vi "DB.indexrange_lua.vi"(5 "LuaVIEW reference":T1) -> (15 "error out":errorcluster)   [LabVIEW 2012]
doc: "Read an index range of values and their corresponding timestamps from a tag's log. Use an index of zero to read from the start of the tag log. By reading a moderate number of values and incrementing the index in a loop, it is possible to efficiently process more values than will fit in memory. To process all values in a log, first use <code>DB.logsize</code> to determine the number of logged values.\n\nBeware that this function may take a while to complete. Because of contention this can happen even when the amount of data being queried is small.\nParameters:\nobj:db, database object.\nstr:tag, name of the tag.\nnum:index, starting index to read from. May not exceed the log size minus the number values being read.\nnum:number, number of values (points or strings) to read as of the specified index.\nResults:\ntab:values, number values, in case of a number tag, or string values, in case of a string tag.\ntab:times, timestamps of the read values.\nErrors:\nTag does not exist.\nDatabases module not initialised.\nCannot read more than \"max points\" values."
uses:
  luaview/typedefs/t_LuaVIEW Reference.ctl
  luaview/subvis/private/LuaVIEW Pull (string).vi
  luaview/subvis/private/LuaVIEW Pull (number).vi
  luaview/subvis/private/LuaVIEW Pull (I32).vi
  luaview/subvis/private/re_LuaVIEW Push (flat data).vi
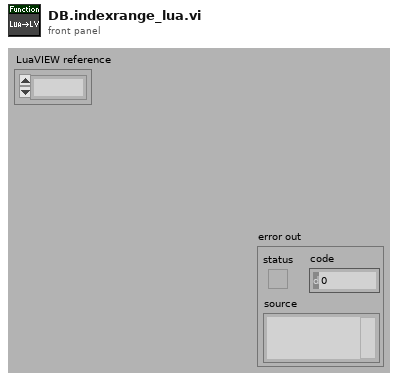
[diagram p1: front panel]
types:
  T1 = typedef "t_LuaVIEW Reference.ctl" = refnum<k1>
  T2 = typedef "t_DataLog Database Info Pane.ctl" = refnum<vi>
  T3 = typedef "t_DataLog Tag Config.ctl" = cluster{"name":string, "unit":string, "temporal":T4, "value":T5, "index":i32, "capacity":i32, "is meta?":bool, "mincapacity":i32, "deadband":dbl, "limit delay":dbl, "format":T6, "precision":u8, "undefine":bool, "update":bool, "update period":u16, "expression":string, "description":string, "logging algorithm":T7, "logging parameters":dbl[]}
  T4 = typedef "t_DataLog Temporal Types.ctl" = enum16{"set&hold", "sample", "event"}
  T5 = typedef "t_DataLog Value Types.ctl" = enum16{"number", "string"}
  T6 = typedef "t_DataLog Numerical Format.ctl" = enum8{"fractional", "exponential", "engineering"}
  T7 = typedef "t_DataLog Logging Algorithms.ctl" = enum16{"nothing", "changes", "everything", "every Nth", "time threshold", "value threshold + prior", "t or v threshold", "t or v threshold + prior"}
  T8 = typedef "t_DataLog Point.ctl" = cluster{"time":dbl, "value":dbl}
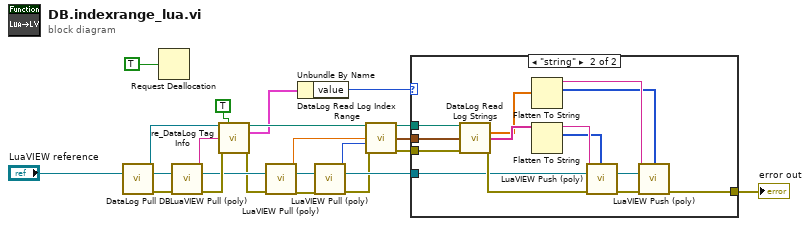
[diagram p0: block diagram]
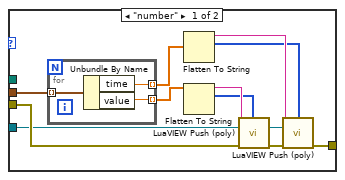
[diagram p2: hidden frame]
diagram:
  n1 = call "DataLog Pull DB.vi"("LuaVIEW reference in"="LuaVIEW reference") -> ("database info"=w1:T2, "LuaVIEW reference out"=w4:T1, "error out"=w2:errorcluster)  [unwired: 12 in]
  n2 = Request Deallocation(TRUE ("flag")) -> ()
  n3 = call-poly "LuaVIEW Pull (poly).vi"("LuaVIEW reference in"=w4, "error in (no error)"=w2) -> ("string"=w5:string, "LuaVIEW reference out"=w9:T1, "error out"=w11:errorcluster)  [unwired: 11 in]
  n4 = call "re_DataLog Tag Info.vi"("database ref (use name)"=w1, "flush? (false)"=TRUE, "tag"=w5, "error in (no error)"=w11) -> ("tag log directory"=w7:path, "tag config"=w6:T3, "error out"=w8:errorcluster)  [unwired: 8 in, 1 out]
  n5 = call-poly "LuaVIEW Pull (poly).vi"("LuaVIEW reference in"=w9, "error in (no error)"=w8) -> ("number"=w14:dbl, "LuaVIEW reference out"=w22:T1, "error out"=w23:errorcluster)  [unwired: 11 in]
  n6 = Unbundle By Name(w6) -> ("value"=w21:T5)
  n7 = call-poly "LuaVIEW Pull (poly).vi"("LuaVIEW reference in"=w22, "error in (no error)"=w23) -> ("I32"=w15:i32, "LuaVIEW reference out"=w20:T1, "error out"=w16:errorcluster)  [unwired: 11 in]
  n8 = call "DataLog Read Log Index Range.vi"("tag log directory"=w7, "log index"=w14, "number of points"=w15, "error in (no error)"=w16) -> ("dup tag log directory"=w19:path, "range of points"=w18:T8[], "error out"=w17:errorcluster)  [unwired: 9 in]
  n9 = case shown="\"string\"" w21 {
    tunnel: w17 -> [w28 w52]
    tunnel: w18 -> [w26 w51]
    tunnel: w19 -> [_ w50]
    tunnel: w20 -> [w27 w48]
    tunnel: [w29 w39] -> w13
    frame "number" {
      n10 = for {
        tunnel: w26 -> [w38] mode=indexing
        tunnel: [w37] -> w25 mode=indexing
        tunnel: [w36] -> w24 mode=indexing
        n11 = Unbundle By Name(w38) -> ("time"=w36:dbl, "value"=w37:dbl)
      }
      n12 = Flatten To String(anything=w24) -> (data string=w31:string, type string=w30:i16[])  [unwired: 3 in, 1 out]
      n13 = Flatten To String(anything=w25) -> (data string=w35:string, type string=w34:i16[])  [unwired: 3 in, 1 out]
      n14 = call-poly "LuaVIEW Push (poly).vi"("flat data"=w35, "type descriptor"=w34, "LuaVIEW reference in"=w27, "error in (no error)"=w28) -> ("LuaVIEW reference out"=w32:T1, "error out"=w33:errorcluster)  [unwired: 10 in]
      n15 = call-poly "LuaVIEW Push (poly).vi"("flat data"=w31, "type descriptor"=w30, "LuaVIEW reference in"=w32, "error in (no error)"=w33) -> ("error out"=w29:errorcluster)  [unwired: 10 in, 1 out]
    }
    frame "string" {
      n16 = call "DataLog Read Log Strings.vi"("tag log directory"=w50, "points (use offsets)"=w51, "error in (no error)"=w52) -> ("times"=w44:dbl[], "strings"=w47:string[], "error out"=w49:errorcluster)  [unwired: 9 in, 1 out]
      n17 = Flatten To String(anything=w44) -> (data string=w41:string, type string=w40:i16[])  [unwired: 3 in, 1 out]
      n18 = Flatten To String(anything=w47) -> (data string=w46:string, type string=w45:i16[])  [unwired: 3 in, 1 out]
      n19 = call-poly "LuaVIEW Push (poly).vi"("flat data"=w46, "type descriptor"=w45, "LuaVIEW reference in"=w48, "error in (no error)"=w49) -> ("LuaVIEW reference out"=w42:T1, "error out"=w43:errorcluster)  [unwired: 10 in]
      n20 = call-poly "LuaVIEW Push (poly).vi"("flat data"=w41, "type descriptor"=w40, "LuaVIEW reference in"=w42, "error in (no error)"=w43) -> ("error out"=w39:errorcluster)  [unwired: 10 in, 1 out]
    }
  }
  "error out" <- w13
